vi "Discover Plugins.vi"() -> (0 "plugins":string[](array[string]))   [LabVIEW 2021, in "Settings.lvlib"]
uses:
  Settings.lvlib
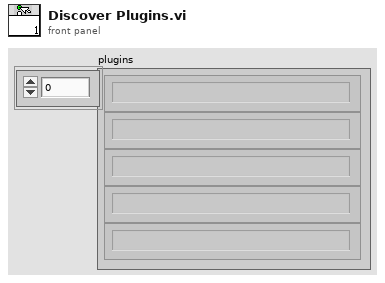
[diagram p1: front panel]
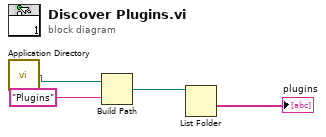
[diagram p0: block diagram]
diagram:
  n1 = call <vilib>:"Application Directory.vi"() -> ("Application Directory"=w4:path)
  n2 = Build Path(base path=w4, name or relative path="Plugins") -> (appended path=w2:path)
  n3 = List Folder(path=w2) -> (folder names=→"plugins":string[])  [unwired: 3 in, 3 out]
